vi "Joystick Deadband.vi"(10 "In":dbl) -> (2 "Out":dbl)   [LabVIEW 2014]
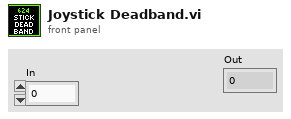
[diagram p1: front panel]
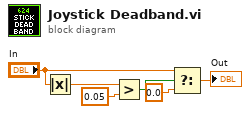
[diagram p0: block diagram]
diagram:
  n1 = Absolute Value(x="In") -> (abs(x)=w6:dbl)
  n2 = Greater?(x=w6, y=0.05) -> (0:w4:bool)
  n3 = Select(t="In", s=w4, f=0.0) -> (s? t:f=→"Out":dbl)
